vi "niDTS Calibration Cal IsNeeded RF Test Close.vi"(0 "Template Tx Test Handle":T1, 11 "error in (no error)":errorcluster) -> (15 "error out":errorcluster)   [LabVIEW 2014, in "niDTS Utilities.lvlib"]
uses:
  niDTS Utilities.lvlib
  Includes/niDTS Calibration Cal IsNeeded RF Test INC Handle.ctl
  Objects/BASE_class/niDTS Calibration Cal IsNeeded RF Test.lvclass
  Framework/Session/Includes/niDTS Session INC Force Destroy.ctl
  Framework/niDTS Framework.lvlib
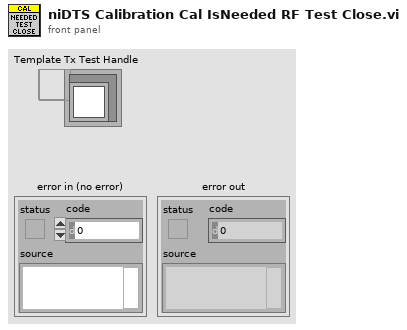
[diagram p1: front panel]
types:
  T1 = typedef "niDTS Utilities.lvlib/niDTS Calibration Cal IsNeeded RF Test INC Handle.ctl" = refnum<data-value>
  T2 = typedef "niDTS Framework.lvlib/niDTS Session INC Force Destroy.ctl" = bool
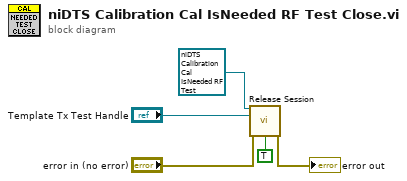
[diagram p0: block diagram]
diagram:
  n1 = call-dynamic "Release Session.vi"("OBJ - Session in"=refnum<class "niDTS Calibration Cal IsNeeded RF Test.lvclass"> refnum ("Template.lvlib:Template Tx Test.lvclass"), "Session Handle in"="Template Tx Test Handle", "error in (no error)"="error in (no error)", "Force Destroy? (F)"=T2 TRUE) -> ("error out"=→"error out":errorcluster)  [unwired: 10 in, 1 out]
